vi "DMM Configure.vi"(4 "Auto Zero":T1=-1 items=["Auto"=-1, "Off"=0, "On"=1, "Once"=2], 6 "Resolution in Digits":T2=5.5 items=["3 1/2"=3.5, "4 1/2"=4.5, "5 1/2"=5.5, "6 1/2"=6.5, "7 1/2"=7.5], 7 "Range":dbl=0.02 format="%.2f", 8 "error in (no error)":errorcluster, 9 "Function":T3, 10 "instrument handle":refnum<k15>, 11 "DMM in":refnum<class "DMM.lvclass">) -> (0 "error out":errorcluster, 2 "instrument handle out":refnum<k15>, 3 "DMM out":refnum<class "DMM.lvclass">)   [LabVIEW 2023, in "HardwareAbstractionLayer_LVOOP.lvlib" / "DMM.lvclass"]
uses:
  DMM.lvclass
  <instrlib>/niDMM/nidmm.llb/niDMM Function.ctl
  <instrlib>/niDMM/nidmm.llb/niDMM Resolution in Digits.ctl
  <instrlib>/niDMM/nidmm.llb/niDMM Auto Zero.ctl
  <instrlib>/niDMM/nidmm.llb/niDMM Configure Measurement Digits.vi
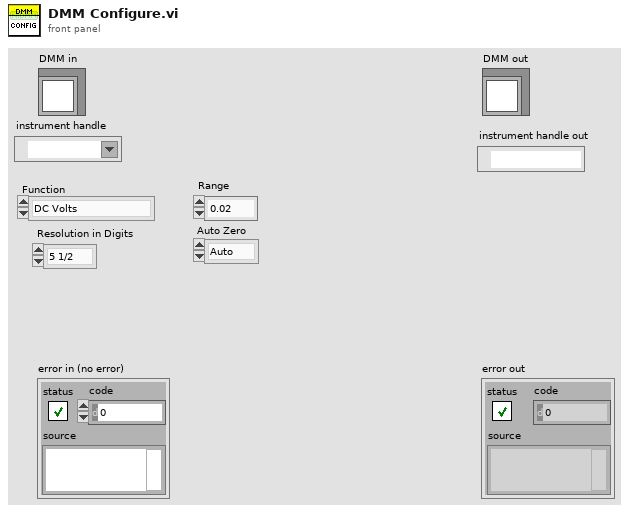
[diagram p1: front panel]
types:
  T1 = typedef "niDMM Auto Zero.ctl" = i32
  T2 = typedef "niDMM Resolution in Digits.ctl" = dbl
  T3 = typedef "niDMM Function.ctl" = enum16{"DC Volts", "AC Volts", "DC Current", "AC Current", "2-wire Resistance", "4-wire Resistance", "Diode", "Frequency", "Period", "AC Volts DC Coupled", "Capacitance", "Inductance", "Temperature"}
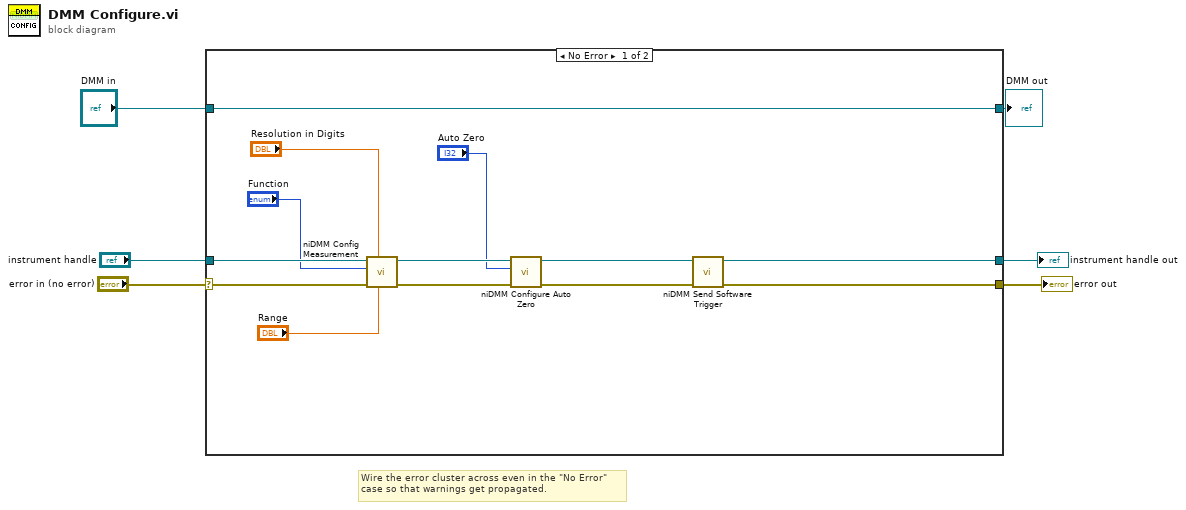
[diagram p0: block diagram]
diagram:
  # "Wire the error cluster across even in the \"No Error\"\ncase so that warnings get propagated."
  n1 = case shown="No Error" "error in (no error)" {
    selector: "error in (no error)" -> [w17 w22]
    tunnel: [w12 w22] -> w5
    tunnel: [w19 w21] -> w3
    tunnel: "DMM in" -> [w19 w21]
    tunnel: "instrument handle" -> [w18 w20]
    tunnel: [w7 w20] -> w1
    frame No Error {
      n2 = call-poly <instrlib>:"niDMM Config Measurement.vi"("Range"="Range", "Resolution in Digits"="Resolution in Digits", "error in (no error)"=w17, "Function"="Function", "instrument handle"=w18) -> ("error out"=w15:errorcluster, "instrument handle out"=w16:refnum<k15>)  [unwired: 5 in]
      n3 = call <instrlib>:"niDMM Configure Auto Zero.vi"("error in (no error)"=w15, "Auto Zero"="Auto Zero", "instrument handle"=w16) -> ("error out"=w14:errorcluster, "instrument handle out"=w13:refnum<k15>)  [unwired: 7 in]
      n4 = call <instrlib>:"niDMM Send Software Trigger.vi"("error in (no error)"=w14, "instrument handle"=w13) -> ("error out"=w12:errorcluster, "instrument handle out"=w7:refnum<k15>)  [unwired: 8 in]
    }
    frame Error {
    }
  }
  "error out" <- w5
  "DMM out" <- w3
  "instrument handle out" <- w1
